vi "D999_Test.vi"() -> ()   [LabVIEW 2018]
panel:
  out "error out":errorcluster
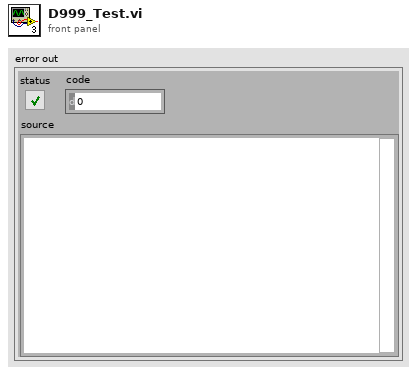
[diagram p1: front panel]
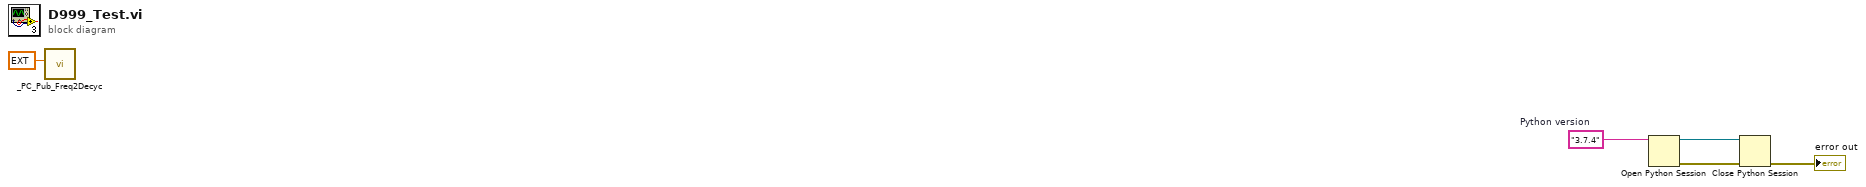
[diagram p0: block diagram]
diagram:
  w4 = "3.7.4"  # Python version
  n1 = call "_PC_Pub_Freq2Decyc.vi"("Freq"=ext 330.0) -> ()  [unwired: 4 in, 5 out]
  n2 = Open Python Session(python version=w4) -> (session out=w3:refnum<k35>, error out=w2:errorcluster)  [unwired: 2 in]
  n3 = Close Python Session(session in=w3, error in=w2) -> (11:→"error out":errorcluster)
